vi "testpath1.vi"() -> (4 "Trajectory":T1[](array[typedef])=[{"t"=0.0, "velocity"=0.0, "acceleration"=6.476596600677185, "pose"={"Translation2d"={"x"=3.048, "y"=5.7912}, "Rotation2d"={"Theta"=0.0}}, "curvature"=0.0}, {"t"=0.17123311369028002, "velocity"=1.1090078020498375, "acceleration"=4.2961846498544, "pose"={"Translation2d"={"x"=3.1429274414869903, "y"=5.789156713424752}, "Rotation2d"={"Theta"=-0.06422251143858711}}, "curvature"=-1.352339474132374}, {"t"=0.20922733042824426, "velocity"=1.2722379727827207, "acceleration"=3.677358730976319, "pose"={"Translation2d"={"x"=3.1879379164245667, "y"=5.784637446231384}, "Rotation2d"={"Theta"=-0.14134128628704262}}, "curvature"=-2.0718634405001795}, {"t"=0.2260059617655958, "velocity"=1.3339390192249632, "acceleration"=2.69992919376837, "pose"={"Translation2d"={"x"=3.2095037093481062, "y"=5.781038434537466}, "Rotation2d"={"Theta"=-0.19076654602166596}}, "curvature"=-2.4518165820756517}, {"t"=0.2417623794212065, "velocity"=1.376480231242554, "acceleration"=1.9121141801744324, "pose"={"Translation2d"={"x"=3.2303501574005176, "y"=5.776413843665275}, "Rotation2d"={"Theta"=-0.2472086209289266}}, "curvature"=-2.8348647690280315}, {"t"=0.25676992707255936, "velocity"=1.4051763759163491, "acceleration"=1.302870542187938, "pose"={"Translation2d"={"x"=3.250421120994618, "y"=5.7706836346877255}, "Rotation2d"={"Theta"=-0.31027843147029727}}, "curvature"=-3.204804579111833}, {"t"=0.2712259317600947, "velocity"=1.4240106785814697, "acceleration"=0.8642938522151383, "pose"={"Translation2d"={"x"=3.2696708581002083, "y"=5.763782592607633}, "Rotation2d"={"Theta"=-0.3793179540434943}}, "curvature"=-3.5390528483466204}, {"t"=0.2852856144456225, "velocity"=1.436162375890667, "acceleration"=0.5888104937887121, "pose"={"Translation2d"={"x"=3.288063591012531, "y"=5.755659708693974}, "Rotation2d"={"Theta"=-0.45334831105890916}}, "curvature"=-3.8111093581327915}, {"t"=0.2990784141416015, "velocity"=1.4442837210903852, "acceleration"=0.467430338613745, "pose"={"Translation2d"={"x"=3.3055730731207307, "y"=5.746277562818135}, "Rotation2d"={"Theta"=-0.5310644010545759}}, "curvature"=-3.9951974468499536}, {"t"=0.31271519881703136, "velocity"=1.450657967968824, "acceleration"=0.47896333266736796, "pose"={"Translation2d"={"x"=3.3221821556763107, "y"=5.735611705790171}, "Rotation2d"={"Theta"=-0.6108919128048625}}, "curvature"=-4.072183097793162}, {"t"=0.3262908218291811, "velocity"=1.4571601936097591, "acceleration"=0.48871790871275284, "pose"={"Translation2d"={"x"=3.3378823545615934, "y"=5.723650041695055}, "Rotation2d"={"Theta"=-0.691106257407233}}, "curvature"=-4.034742483694034}, {"t"=0.33989122988519443, "velocity"=1.463806956592534, "acceleration"=0.6389634123631391, "pose"={"Translation2d"={"x"=3.3526734170581807, "y"=5.710392210228935}, "Rotation2d"={"Theta"=-0.7699910385979648}}, "curvature"=-3.889545372820958}, {"t"=0.3535886216760073, "velocity"=1.4725590887916666, "acceleration"=0.9100004128758293, "pose"={"Translation2d"={"x"=3.3665628886154106, "y"=5.695848969035388}, "Rotation2d"={"Theta"=-0.8459976247266188}}, "curvature"=-3.655429411840859}, {"t"=0.36742916395811687, "velocity"=1.4851539879828117, "acceleration"=1.279346026685717, "pose"={"Translation2d"={"x"=3.379565679618818, "y"=5.680041576041672}, "Rotation2d"={"Theta"=-0.9178671856268694}}, "curvature"=-3.3584701883490546}, {"t"=0.3814317421588926, "velocity"=1.5030681307673301, "acceleration"=1.7224519652606627, "pose"={"Translation2d"={"x"=3.3917036321585923, "y"=5.663001171794983}, "Rotation2d"={"Theta"=-0.9846923785837841}}, "curvature"=-3.0261374552775786}, {"t"=0.3955886938394116, "velocity"=1.5274528000115404, "acceleration"=2.2139912769151002, "pose"={"Translation2d"={"x"=3.403005086798038, "y"=5.644768161798704}, "Rotation2d"={"Theta"=-1.045917898803563}}, "curvature"=-2.682615762850822}, {"t"=0.4098690549978487, "velocity"=1.5590693950475174, "acceleration"=2.7295239699549225, "pose"={"Translation2d"={"x"=3.413504449342032, "y"=5.625391598848665}, "Rotation2d"={"Theta"=-1.1012958170019365}}, "curvature"=-2.3462802984426165}, {"t"=0.4242240484064563, "velocity"=1.5982516936448568, "acceleration"=3.2472177401001474, "pose"={"Translation2d"={"x"=3.4232417576054854, "y"=5.604928565369393}, "Rotation2d"={"Theta"=-1.1508176245777009}}, "curvature"=-2.0291930867365533}, {"t"=0.4385938505454666, "velocity"=1.6449135700723803, "acceleration"=3.749276185877941, "pose"={"Translation2d"={"x"=3.432262248181799, "y"=5.583443555750367}, "Rotation2d"={"Theta"=-1.194641984554156}}, "curvature"=-1.7378998404999786}, {"t"=0.467145646075665, "velocity"=1.7519621371178093, "acceleration"=4.698691157555746, "pose"={"Translation2d"={"x"=3.448357117149824, "y"=5.537698939493257}, "Rotation2d"={"Theta"=-1.2662953329622}}, "curvature"=-1.2393449917060648}, {"t"=0.49511151459182356, "velocity"=1.8833651162280503, "acceleration"=5.481491834882887, "pose"={"Translation2d"={"x"=3.462238461764593, "y"=5.488798473269863}, "Rotation2d"={"Theta"=-1.3187509615342337}}, "curvature"=-0.8420823071385931}, {"t"=0.5220677486425962, "velocity"=2.0311254930765528, "acceleration"=6.1297774268358065, "pose"={"Translation2d"={"x"=3.4744111411818324, "y"=5.437461941232202}, "Rotation2d"={"Theta"=-1.3543922510428046}}, "curvature"=-0.5209865526831502}, {"t"=0.5719547077588071, "velocity"=2.3369214489605827, "acceleration"=2.469114644942459, "pose"={"Translation2d"={"x"=3.4958440287769785, "y"=5.3306365296803655}, "Rotation2d"={"Theta"=-1.3817968158575638}}, "curvature"=-9.126528454248283e-16}, {"t"=0.617482683655318, "velocity"=2.4493352410012452, "acceleration"=1.7489716291390172, "pose"={"Translation2d"={"x"=3.517276916372125, "y"=5.223811118128529}, "Rotation2d"={"Theta"=-1.3543922510428048}}, "curvature"=0.5209865526831473}, {"t"=0.6388600471608528, "velocity"=2.4867236432782174, "acceleration"=-4.5602342650468595, "pose"={"Translation2d"={"x"=3.529449595789364, "y"=5.172474586090868}, "Rotation2d"={"Theta"=-1.3187509615342345}}, "curvature"=0.8420823071385926}, {"t"=0.6596998334639634, "velocity"=2.3916893357025177, "acceleration"=-10.000000000000014, "pose"={"Translation2d"={"x"=3.5433309404041333, "y"=5.123574119867473}, "Rotation2d"={"Theta"=-1.2662953329621998}}, "curvature"=1.2393449917060613}, {"t"=0.6809167339585578, "velocity"=2.1795203307565743, "acceleration"=-9.999999999999991, "pose"={"Translation2d"={"x"=3.5594258093721582, "y"=5.077829503610364}, "Rotation2d"={"Theta"=-1.1946419845541556}}, "curvature"=1.7378998404999833}, {"t"=0.6918839260254118, "velocity"=2.069848410088034, "acceleration"=-10.00000000000002, "pose"={"Translation2d"={"x"=3.568446299948472, "y"=5.056344493991338}, "Rotation2d"={"Theta"=-1.1508176245777002}}, "curvature"=2.0291930867365586}, {"t"=0.7031383604394913, "velocity"=1.9573040659472387, "acceleration"=-9.99999999999999, "pose"={"Translation2d"={"x"=3.5781836082119254, "y"=5.035881460512066}, "Rotation2d"={"Theta"=-1.1012958170019373}}, "curvature"=2.34628029844261}, {"t"=0.7147418355471609, "velocity"=1.8412693148705435, "acceleration"=-8.783912356688163, "pose"={"Translation2d"={"x"=3.5886829707559196, "y"=5.016504897562027}, "Rotation2d"={"Theta"=-1.0459178988035625}}, "curvature"=2.6826157628508227}, {"t"=0.7267353138837706, "velocity"=1.7359196523099263, "acceleration"=-7.356386910661949, "pose"={"Translation2d"={"x"=3.5999844253953652, "y"=4.998271887565748}, "Rotation2d"={"Theta"=-0.984692378583783}}, "curvature"=3.026137455277591}, {"t"=0.739111944458336, "velocity"=1.6448723691530953, "acceleration"=-5.785266152459879, "pose"={"Translation2d"={"x"=3.612122377935139, "y"=4.981231483319059}, "Rotation2d"={"Theta"=-0.9178671856268704}}, "curvature"=3.358470188349063}, {"t"=0.7518404874903905, "velocity"=1.5712343599796215, "acceleration"=-4.1137462458469605, "pose"={"Translation2d"={"x"=3.6251251689385464, "y"=4.965424090325343}, "Rotation2d"={"Theta"=-0.8459976247266192}}, "curvature"=3.6554294118408754}, {"t"=0.7648614683812988, "velocity"=1.5176693487224022, "acceleration"=-2.3761113788041133, "pose"={"Translation2d"={"x"=3.639014640495776, "y"=4.950880849131797}, "Rotation2d"={"Theta"=-0.7699910385979658}}, "curvature"=3.889545372820968}, {"t"=0.7780863251520889, "velocity"=1.4862456160662731, "acceleration"=-0.5927648597672066, "pose"={"Translation2d"={"x"=3.653805702992363, "y"=4.937623017665676}, "Rotation2d"={"Theta"=-0.6911062574072322}}, "curvature"=4.034742483694059}, {"t"=0.7914019384076868, "velocity"=1.4783525884421043, "acceleration"=0.318594910695986, "pose"={"Translation2d"={"x"=3.6695059018776464, "y"=4.92566135357056}, "Rotation2d"={"Theta"=-0.6108919128048621}}, "curvature"=4.07218309779317}, {"t"=0.8047347057336984, "velocity"=1.4826003402576653, "acceleration"=0.39202796582971616, "pose"={"Translation2d"={"x"=3.6861149844332273, "y"=4.914995496542596}, "Rotation2d"={"Theta"=-0.5310644010545743}}, "curvature"=3.995197446849954}, {"t"=0.8181096139300382, "velocity"=1.4878436783110356, "acceleration"=0.6050898214304106, "pose"={"Translation2d"={"x"=3.7036244665414264, "y"=4.905613350666757}, "Rotation2d"={"Theta"=-0.45334831105891005}}, "curvature"=3.8111093581327915}, {"t"=0.8315865754564393, "velocity"=1.4959984505544701, "acceleration"=0.9427956080909262, "pose"={"Translation2d"={"x"=3.7220171994537488, "y"=4.897490466753097}, "Rotation2d"={"Theta"=-0.3793179540434954}}, "curvature"=3.539052848346631}, {"t"=0.8451975787127834, "velocity"=1.5088308446462626, "acceleration"=1.3877862387284934, "pose"={"Translation2d"={"x"=3.74126693655934, "y"=4.890589424673006}, "Rotation2d"={"Theta"=-0.3102784314702983}}, "curvature"=3.2048045791118343}, {"t"=0.8589445083496284, "velocity"=1.527908644421045, "acceleration"=1.9216925627443424, "pose"={"Translation2d"={"x"=3.76133790015344, "y"=4.884859215695456}, "Rotation2d"={"Theta"=-0.2472086209289246}}, "curvature"=2.834864769028038}, {"t"=0.8727992700534354, "velocity"=1.554533236945846, "acceleration"=2.5272605993081534, "pose"={"Translation2d"={"x"=3.782184348205851, "y"=4.880234624823265}, "Rotation2d"={"Theta"=-0.19076654602166704}}, "curvature"=2.4518165820756592}, {"t"=0.8867067454783021, "velocity"=1.589681051622958, "acceleration"=3.1912034533747446, "pose"={"Translation2d"={"x"=3.803750141129391, "y"=4.876635613129347}, "Rotation2d"={"Theta"=-0.14134128628704148}}, "curvature"=2.0718634405001946}, {"t"=0.9143938315284367, "velocity"=1.678036176240031, "acceleration"=4.73942738227151, "pose"={"Translation2d"={"x"=3.848760616066967, "y"=4.8721163459359795}, "Rotation2d"={"Theta"=-0.06422251143858412}}, "curvature"=1.3523394741323758}, {"t"=0.96706039361214, "velocity"=1.9276455227096372, "acceleration"=3.0715111325660827, "pose"={"Translation2d"={"x"=3.9436880575539566, "y"=4.870073059360731}, "Rotation2d"={"Theta"=0.0}}, "curvature"=-5.978347474406742e-15}, {"t"=0.9914069633882024, "velocity"=2.00242628281661, "acceleration"=-9.866558396704047, "pose"={"Translation2d"={"x"=3.9915282859876635, "y"=4.870471030718632}, "Rotation2d"={"Theta"=0.02489796257300611}}, "curvature"=1.0424449028682865}, {"t"=1.0158542397991215, "velocity"=1.7612158024679117, "acceleration"=-10.0, "pose"={"Translation2d"={"x"=4.0374581515948575, "y"=4.873106215628532}, "Rotation2d"={"Theta"=0.09874992223341753}}, "curvature"=2.224603541642049}, {"t"=1.028773099528808, "velocity"=1.6320272051710467, "acceleration"=-10.00000000000001, "pose"={"Translation2d"={"x"=4.059203777534808, "y"=4.875852973414197}, "Rotation2d"={"Theta"=0.15517703568404698}}, "curvature"=2.945325833594567}, {"t"=1.0422492212162193, "velocity"=1.497265988296933, "acceleration"=-9.999999999999995, "pose"={"Translation2d"={"x"=4.079913590385775, "y"=4.879814840732562}, "Rotation2d"={"Theta"=0.22576892383844907}}, "curvature"=3.771975109233371}, {"t"=1.0564478600345162, "velocity"=1.3552796001139649, "acceleration"=-10.0, "pose"={"Translation2d"={"x"=4.099447291916161, "y"=4.8851573927805925}, "Rotation2d"={"Theta"=0.31127512742411795}}, "curvature"=4.687301631551826}, {"t"=1.0639098158850877, "velocity"=1.2806600416082508, "acceleration"=-8.960349793118844, "pose"={"Translation2d"={"x"=4.108734904396276, "y"=4.88839162423552}, "Rotation2d"={"Theta"=0.3596963482392804}}, "curvature"=5.1604774227139325}, {"t"=1.0716619724847825, "velocity"=1.2111980068239518, "acceleration"=-7.37204937958643, "pose"={"Translation2d"={"x"=4.11768515490125, "y"=4.892022365594454}, "Rotation2d"={"Theta"=0.4118045814451839}}, "curvature"=5.627208208212191}, {"t"=1.0797049284054525, "velocity"=1.1519049386189353, "acceleration"=-5.8501010886108675, "pose"={"Translation2d"={"x"=4.126286161110897, "y"=4.896063759420438}, "Rotation2d"={"Theta"=0.46741393974564627}}, "curvature"=6.070143300819135}, {"t"=1.0880171770797658, "velocity"=1.1032774436005313, "acceleration"=-4.3931111257363895, "pose"={"Translation2d"={"x"=4.134527226860072, "y"=4.900528572940315}, "Rotation2d"={"Theta"=0.5262247253095962}}, "curvature"=6.4689371688986705}, {"t"=1.0965666833417067, "velocity"=1.065718512521646, "acceleration"=-2.9947614126980446, "pose"={"Translation2d"={"x"=4.142398817255443, "y"=4.9054282266975635}, "Rotation2d"={"Theta"=0.5878142703411942}}, "curvature"=6.801867933374289}, {"t"=1.1053108923698223, "velocity"=1.0395316927396794, "acceleration"=-1.644038700543018, "pose"={"Translation2d"={"x"=4.149892533792267, "y"=4.910772823205141}, "Rotation2d"={"Theta"=0.6516384264173147}}, "curvature"=7.0482280881810375}, {"t"=1.114197959309006, "velocity"=1.024921010757345, "acceleration"=-0.3264829679038617, "pose"={"Translation2d"={"x"=4.157001089471175, "y"=4.916571175598313}, "Rotation2d"={"Theta"=0.7170462810626088}}, "curvature"=7.191153782485671}, {"t"=1.1231692479249908, "velocity"=1.021992037824076, "acceleration"=0.2202461473454793, "pose"={"Translation2d"={"x"=4.163718283914939, "y"=4.922830836287498}, "Rotation2d"={"Theta"=0.7833085290546009}}, "curvature"=7.220297530496624}, {"t"=1.1321926352252907, "velocity"=1.0239794041129733, "acceleration"=0.2613386516886456, "pose"={"Translation2d"={"x"=4.170038978485256, "y"=4.929558125611102}, "Rotation2d"={"Theta"=0.8496570437914189}}, "curvature"=7.133648349381659}, {"t"=1.1412851720405306, "velocity"=1.0263556354246974, "acceleration"=0.36975176742313487, "pose"={"Translation2d"={"x"=4.175959071399523, "y"=4.936758160488354}, "Rotation2d"={"Theta"=0.9153304525826212}}, "curvature"=6.937963941560547}, {"t"=1.1504803823584737, "velocity"=1.0297555806915843, "acceleration"=0.5404530754500246, "pose"={"Translation2d"={"x"=4.181475472847611, "y"=4.944434883072148}, "Rotation2d"={"Theta"=0.9796189350625144}}, "curvature"=6.647673983564364}, {"t"=1.1598045158588555, "velocity"=1.0347948373177722, "acceleration"=0.7676723372075956, "pose"={"Translation2d"={"x"=4.186586080108644, "y"=4.952591089401876}, "Rotation2d"={"Theta"=1.0419016817560647}}, "curvature"=6.2825755962054215}, {"t"=1.1692756134126592, "velocity"=1.0420655369128218, "acceleration"=1.0448100439943895, "pose"={"Translation2d"={"x"=4.191289752667781, "y"=4.961228458056268}, "Rotation2d"={"Theta"=1.1016723796168877}}, "curvature"=5.864961617895575}, {"t"=1.1789028252260947, "velocity"=1.0521241445111607, "acceleration"=1.3644206978494995, "pose"={"Translation2d"={"x"=4.195586287332981, "y"=4.970347578806229}, "Rotation2d"={"Theta"=1.158550959080056}}, "curvature"=5.416876643870572}, {"t"=1.1886861818206726, "velocity"=1.065472758743245, "acceleration"=1.7182932416672998, "pose"={"Translation2d"={"x"=4.199476393351792, "y"=4.979947981267677}, "Rotation2d"={"Theta"=1.2122826165113503}}, "curvature"=4.95801139300344}, {"t"=1.1986169596194587, "velocity"=1.082536747119399, "acceleration"=2.097635180915759, "pose"={"Translation2d"={"x"=4.202961667528121, "y"=4.99002816355438}, "Rotation2d"={"Theta"=1.262727036042975}}, "curvature"=4.504453400761753}, {"t"=1.2086786887623995, "velocity"=1.1036425841504771, "acceleration"=2.4933470970556573, "pose"={"Translation2d"={"x"=4.206044569339014, "y"=5.000585620930793}, "Rotation2d"={"Theta"=1.3098414998752301}}, "curvature"=4.068249389336106}, {"t"=1.2188487341307996, "velocity"=1.1290000372467017, "acceleration"=2.8963564023842063, "pose"={"Translation2d"={"x"=4.208728396051428, "y"=5.011616874464897}, "Rotation2d"={"Theta"=1.353661372079742}}, "curvature"=3.657578496396842}, {"t"=1.2394185064788306, "velocity"=1.1885774290825064, "acceleration"=3.713919348923273, "pose"={"Translation2d"={"x"=4.212916052898901, "y"=5.035082155212745}, "Rotation2d"={"Theta"=1.4318344499836884}}, "curvature"=2.929601338458617}, {"t"=1.2601460788316914, "velocity"=1.2655579611000036, "acceleration"=4.461275386160614, "pose"={"Translation2d"={"x"=4.215566826442033, "y"=5.060377779220092}, "Rotation2d"={"Theta"=1.4984049289713866}}, "curvature"=2.3317640084834035}, {"t"=1.2808006503422769, "velocity"=1.357703692591873, "acceleration"=5.095839652765746, "pose"={"Translation2d"={"x"=4.216734717164677, "y"=5.0874437665471035}, "Rotation2d"={"Theta"=1.55478349765767}}, "curvature"=1.8531035101655093}, {"t"=1.3012055233982476, "velocity"=1.4616836538201397, "acceleration"=5.595908452038135, "pose"={"Translation2d"={"x"=4.216484741399902, "y"=5.116207300782747}, "Rotation2d"={"Theta"=1.6023775716018394}}, "curvature"=1.4744007975298525}, {"t"=1.340899235076796, "velocity"=1.6838060304948936, "acceleration"=6.230746263692941, "pose"={"Translation2d"={"x"=4.212041557407635, "y"=5.178477063324598}, "Rotation2d"={"Theta"=1.6761501755710626}}, "curvature"=0.9392024761393751}, {"t"=1.378914127577943, "velocity"=1.920667179911104, "acceleration"=6.2335527791056595, "pose"={"Translation2d"={"x"=4.202947464114885, "y"=5.2463826479837765}, "Rotation2d"={"Theta"=1.7278375836964097}}, "curvature"=0.5985723564344896}, {"t"=1.4151685277805834, "velocity"=2.1466608970490815, "acceleration"=5.972100041045658, "pose"={"Translation2d"={"x"=4.190037943917913, "y"=5.318972933370419}, "Rotation2d"={"Theta"=1.762972431133745}}, "curvature"=0.37085109413942363}, {"t"=1.4497582613554434, "velocity"=2.353234246351261, "acceleration"=5.715153823531552, "pose"={"Translation2d"={"x"=4.174248291539145, "y"=5.395179436072257}, "Rotation2d"={"Theta"=1.7851143940198193}}, "curvature"=0.20712333589779897}, {"t"=1.4827014188040084, "velocity"=2.5415094586026297, "acceleration"=4.991596402415036, "pose"={"Translation2d"={"x"=4.15658813360673, "y"=5.473845651160227}, "Rotation2d"={"Theta"=1.7964066262000233}}, "curvature"=0.07732682064803718}, {"t"=1.5140101743888579, "velocity"=2.6977901303440555, "acceleration"=3.462433098634447, "pose"={"Translation2d"={"x"=4.138115948234097, "y"=5.553756392694062}, "Rotation2d"={"Theta"=1.797941459001904}}, "curvature"=-0.03890299722649509}, {"t"=1.5438194895916852, "velocity"=2.801002889949952, "acceleration"=2.28358192418938, "pose"={"Translation2d"={"x"=4.119913584599508, "y"=5.633667134227898}, "Rotation2d"={"Theta"=1.7899526357701192}}, "curvature"=-0.15806528232633305}, {"t"=1.5722131258219068, "velocity"=2.8658420844072947, "acceleration"=1.1280911880608837, "pose"={"Translation2d"={"x"=4.103060782525623, "y"=5.712333349315868}, "Rotation2d"={"Theta"=1.7718643564217582}}, "curvature"=-0.29715897337264985}, {"t"=1.5991356675412876, "velocity"=2.8962131664811297, "acceleration"=-9.20556998883836, "pose"={"Translation2d"={"x"=4.088609692059048, "y"=5.788539852017706}, "Rotation2d"={"Theta"=1.7422093760368393}}, "curvature"=-0.47809899701639796}, {"t"=1.6256014382911395, "velocity"=2.652580661534816, "acceleration"=-10.0, "pose"={"Translation2d"={"x"=4.077559393049899, "y"=5.861130137404348}, "Rotation2d"={"Theta"=1.6984091663283192}}, "curvature"=-0.7335651483582837}, {"t"=1.6527120542126659, "velocity"=2.3814745023195516, "acceleration"=-10.0, "pose"={"Translation2d"={"x"=4.070830414731352, "y"=5.929035722063526}, "Rotation2d"={"Theta"=1.6364062011238778}}, "curvature"=-1.1154107963944244}, {"t"=1.6804879513106363, "velocity"=2.1037155313398475, "acceleration"=-10.0, "pose"={"Translation2d"={"x"=4.069239255299209, "y"=5.991305484605376}, "Rotation2d"={"Theta"=1.5502007632830788}}, "curvature"=-1.704292909703093}, {"t"=1.6946526330139349, "velocity"=1.9620687143068627, "acceleration"=-10.0, "pose"={"Translation2d"={"x"=4.0705907967927235, "y"=6.02006901884102}, "Rotation2d"={"Theta"=1.4955417572753067}}, "curvature"=-2.109636818268285}, {"t"=1.7090537412581592, "velocity"=1.818057631864618, "acceleration"=-10.0, "pose"={"Translation2d"={"x"=4.073472901491444, "y"=6.047135006168031}, "Rotation2d"={"Theta"=1.4316285292429842}}, "curvature"=-2.6066526422178895}, {"t"=1.7237796290608398, "velocity"=1.670798753837812, "acceleration"=-10.000000000000009, "pose"={"Translation2d"={"x"=4.077947026190856, "y"=6.072430630175378}, "Rotation2d"={"Theta"=1.3572912194315836}}, "curvature"=-3.201603995245795}, {"t"=1.7389851361347335, "velocity"=1.5187436830988745, "acceleration"=-9.737411955646257, "pose"={"Translation2d"={"x"=4.084063348167772, "y"=6.095895910923225}, "Rotation2d"={"Theta"=1.2715767469971895}}, "curvature"=-3.8846875040570623}, {"t"=1.746841231086964, "velocity"=1.4422456501863328, "acceleration"=-8.693525280628265, "pose"={"Translation2d"={"x"=4.08774973333553, "y"=6.106927164457329}, "Rotation2d"={"Theta"=1.2242916335995968}}, "curvature"=-4.248681733504786}, {"t"=1.7548919186475858, "velocity"=1.3722567943516293, "acceleration"=-7.573674503844255, "pose"={"Translation2d"={"x"=4.091859968917197, "y"=6.117484621833742}, "Rotation2d"={"Theta"=1.1740721589970857}}, "curvature"=-4.6172536318928925}, {"t"=1.7631348285275343, "velocity"=1.3098276779563764, "acceleration"=-6.402583044036974, "pose"={"Translation2d"={"x"=4.09639680012182, "y"=6.127564804120445}, "Rotation2d"={"Theta"=1.121021538191881}}, "curvature"=-4.979251146157832}, {"t"=1.7715601144787159, "velocity"=1.2558840849841792, "acceleration"=-5.201361462476047, "pose"={"Translation2d"={"x"=4.101362117889191, "y"=6.137165206581893}, "Rotation2d"={"Theta"=1.065331019761457}}, "curvature"=-5.321029145184125}, {"t"=1.780149495611209, "velocity"=1.2112076089751114, "acceleration"=-3.9857019909796154, "pose"={"Translation2d"={"x"=4.106756934006624, "y"=6.146284327331855}, "Rotation2d"={"Theta"=1.0072891796544916}}, "curvature"=-5.627139989619832}, {"t"=1.7888758551769213, "velocity"=1.1764269402800478, "acceleration"=-2.7649783583485377, "pose"={"Translation2d"={"x"=4.1125813562257285, "y"=6.154921695986246}, "Rotation2d"={"Theta"=0.9472849671677978}}, "curvature"=-5.881543048589161}, {"t"=1.7977036043272625, "velocity"=1.1520184049264248, "acceleration"=-1.5423141829814615, "pose"={"Translation2d"={"x"=4.118834563379194, "y"=6.163077902315973}, "Rotation2d"={"Theta"=0.8858023370442392}}, "curvature"=-6.069252134391077}, {"t"=1.8065899293433723, "velocity"=1.1383128998194958, "acceleration"=-0.3155220941942261, "pose"={"Translation2d"={"x"=4.125514780497557, "y"=6.170754624899767}, "Rotation2d"={"Theta"=0.8234052766792812}}, "curvature"=-6.178180734930033}, {"t"=1.8154868927870538, "velocity"=1.135505711281776, "acceleration"=0.24470910627744785, "pose"={"Translation2d"={"x"=4.132619253925988, "y"=6.1779546597770185}, "Rotation2d"={"Theta"=0.7607136230550819}}, "curvature"=-6.200816154801577}, {"t"=1.8243675118425575, "velocity"=1.1376788796340387, "acceleration"=0.28113639026863074, "pose"={"Translation2d"={"x"=4.14014422644106, "y"=6.184681949100622}, "Rotation2d"={"Theta"=0.6983719203264055}}, "curvature"=-6.135325080865791}, {"t"=1.8332454071558555, "velocity"=1.140174779075602, "acceleration"=0.38126460611539575, "pose"={"Translation2d"={"x"=4.148084912367533, "y"=6.190941609789808}, "Rotation2d"={"Theta"=0.6370151468553518}}, "curvature"=-5.985803301665135}, {"t"=1.842148555066692, "velocity"=1.1435692342570143, "acceleration"=0.5407623442436613, "pose"={"Translation2d"={"x"=4.156435472695123, "y"=6.19673996218298}, "Rotation2d"={"Theta"=0.5772358957348409}}, "curvature"=-5.761605026760297}, {"t"=1.851098167850816, "velocity"=1.1484088478462302, "acceleration"=0.7547803531836187, "pose"={"Translation2d"={"x"=4.165188990195285, "y"=6.202084558690557}, "Rotation2d"={"Theta"=0.5195572459232708}}, "curvature"=-5.4759355108304035}, {"t"=1.8601082548048984, "velocity"=1.1552094844596477, "acceleration"=1.0179693969022292, "pose"={"Translation2d"={"x"=4.174337444537986, "y"=6.206984212447806}, "Rotation2d"={"Theta"=0.4644142421097831}}, "curvature"=-5.144063402158328}, {"t"=1.8691853505867588, "velocity"=1.1644496901783319, "acceleration"=1.3245465878706673, "pose"={"Translation2d"={"x"=4.183871687408488, "y"=6.211449025967683}, "Rotation2d"={"Theta"=0.412145081774197}}, "curvature"=-4.781547922652296}, {"t"=1.8783285252781927, "velocity"=1.176560251018176, "acceleration"=1.6684210160405477, "pose"={"Translation2d"={"x"=4.193781417624111, "y"=6.215490419793666}, "Rotation2d"={"Theta"=0.3629913658889686}}, "curvature"=-4.402790490829444}, {"t"=1.8875297493649963, "velocity"=1.1919117666578978, "acceleration"=2.0433809727929386, "pose"={"Translation2d"={"x"=4.204055156251034, "y"=6.219121161152601}, "Rotation2d"={"Theta"=0.3171055417051797}}, "curvature"=-4.020070233256811}, {"t"=1.896774632488839, "velocity"=1.2108025849288526, "acceleration"=2.4433351653567836, "pose"={"Translation2d"={"x"=4.214680221721041, "y"=6.222355392607528}, "Rotation2d"={"Theta"=0.2745631182576509}}, "curvature"=-3.6430758192368002}, {"t"=1.9153238024935424, "velocity"=1.2561244242895255, "acceleration"=3.3185049010554564, "pose"={"Translation2d"={"x"=4.236927444446259, "y"=6.227697944655556}, "Rotation2d"={"Theta"=0.19951401475255184}}, "curvature"=-2.93198664532826}, {"t"=1.933820056584235, "velocity"=1.317504334140656, "acceleration"=4.233901957263671, "pose"={"Translation2d"={"x"=4.2603966350040565, "y"=6.231659811973921}, "Rotation2d"={"Theta"=0.137466626331804}}, "curvature"=-2.298899890179479}, {"t"=1.9520324579136425, "velocity"=1.394613855775706, "acceleration"=5.173993769155555, "pose"={"Translation2d"={"x"=4.284940507922383, "y"=6.234406569759586}, "Rotation2d"={"Theta"=0.08770188039099987}}, "curvature"=-1.7466793480593512}, {"t"=1.986842242857437, "velocity"=1.574719466180544, "acceleration"=7.330345470662451, "pose"={"Translation2d"={"x"=4.336554207991923, "y"=6.237041754669483}, "Rotation2d"={"Theta"=0.022203649613225084}}, "curvature"=-0.8277745333865666}, {"t"=2.0185360873473095, "velocity"=1.807046295584759, "acceleration"=4.2458080152074125, "pose"={"Translation2d"={"x"=4.390143309352523, "y"=6.237439726027385}, "Rotation2d"={"Theta"=-2.4698950781383874e-14}}, "curvature"=-3.815788435761329e-14}, {"t"=2.0472272524369703, "velocity"=1.9288634742880806, "acceleration"=1.0486386048007321, "pose"={"Translation2d"={"x"=4.443735509762219, "y"=6.237025399682183}, "Rotation2d"={"Theta"=-0.023111687763194597}}, "curvature"=-0.8612687529609949}, {"t"=2.073842875827728, "velocity"=1.9567736444664663, "acceleration"=-9.999999999999991, "pose"={"Translation2d"={"x"=4.4953720067862015, "y"=6.234281919502013}, "Rotation2d"={"Theta"=-0.09121412756685161}}, "curvature"=-1.812232090926253}, {"t"=2.086920837778034, "velocity"=1.8259940249634075, "acceleration"=-10.0, "pose"={"Translation2d"={"x"=4.519941596714094, "y"=6.231422281259404}, "Rotation2d"={"Theta"=-0.142853118425267}}, "curvature"=-2.3779640775710726}, {"t"=2.100496514207632, "velocity"=1.6902372606674274, "acceleration"=-9.999999999999991, "pose"={"Translation2d"={"x"=4.543450100441191, "y"=6.227297597475901}, "Rotation2d"={"Theta"=-0.20706951595517584}}, "curvature"=-3.018514929278512}, {"t"=2.1146921792792663, "velocity"=1.5482806099510837, "acceleration"=-10.0, "pose"={"Translation2d"={"x"=4.565753467284166, "y"=6.22173548849439}, "Rotation2d"={"Theta"=-0.2844362355914516}}, "curvature"=-3.7245183081897935}, {"t"=2.1220895634622585, "velocity"=1.4743067681211628, "acceleration"=-9.504526862324147, "pose"={"Translation2d"={"x"=4.576413966244121, "y"=6.218368343418026}, "Rotation2d"={"Theta"=-0.3281202672351931}}, "curvature"=-4.091529876288796}, {"t"=2.129728946931762, "velocity"=1.4016980427236734, "acceleration"=-8.087405720691313, "pose"={"Translation2d"={"x"=4.5867286223244506, "y"=6.214588393510095}, "Rotation2d"={"Theta"=-0.3750828671061514}}, "curvature"=-4.457726587962087}, {"t"=2.137620002566903, "velocity"=1.3378798742377402, "acceleration"=-6.693809188303754, "pose"={"Translation2d"={"x"=4.596685195736315, "y"=6.210380915006331}, "Rotation2d"={"Theta"=-0.4251998875483632}}, "curvature"=-4.812409856452728}, {"t"=2.1457493159332444, "velocity"=1.2834638017315259, "acceleration"=-5.329606742238304, "pose"={"Translation2d"={"x"=4.606272656428732, "y"=6.205732615999336}, "Rotation2d"={"Theta"=-0.4782652371070451}}, "curvature"=-5.142699077935643}, {"t"=2.1540959506136557, "velocity"=1.2389795212638062, "acceleration"=-3.997720046989495, "pose"={"Translation2d"={"x"=4.6154811587767215, "y"=6.200631606608227}, "Rotation2d"={"Theta"=-0.5339817257639918}}, "curvature"=-5.434258292036248}, {"t"=2.1626310516406835, "velocity"=1.2048585767849769, "acceleration"=-2.697479414591349, "pose"={"Translation2d"={"x"=4.624302016269438, "y"=6.195067369148284}, "Rotation2d"={"Theta"=-0.5919579383647916}}, "curvature"=-5.672484092954958}, {"t"=2.1713181813400104, "velocity"=1.1814252232491569, "acceleration"=-1.4248404756467294, "pose"={"Translation2d"={"x"=4.6327276761983205, "y"=6.189030728300598}, "Rotation2d"={"Theta"=-0.6517131706679116}}, "curvature"=-5.844061494250866}, {"t"=2.180114497827897, "velocity"=1.168891875480618, "acceleration"=-0.17336165892091332, "pose"={"Translation2d"={"x"=4.640751694345225, "y"=6.18251382128172}, "Rotation2d"={"Theta"=-0.7126915500305057}}, "curvature"=-5.938653506639202}, {"t"=2.18897274812823, "velocity"=1.1673561945134154, "acceleration"=0.2515730993059894, "pose"={"Translation2d"={"x"=4.648368709670568, "y"=6.175510068013311}, "Rotation2d"={"Theta"=-0.7742849819238307}}, "curvature"=-5.950383323266472}, {"t"=2.1978712246817467, "velocity"=1.1695948118390853, "acceleration"=0.2953139623870331, "pose"={"Translation2d"={"x"=4.655574419001469, "y"=6.1680141412917875}, "Rotation2d"={"Theta"=-0.8358628259916795}}, "curvature"=-5.878755435370926}, {"t"=2.2068281686357123, "velocity"=1.1722399224490094, "acceleration"=0.40175171275952587, "pose"={"Translation2d"={"x"=4.662365551719884, "y"=6.160021936957975}, "Rotation2d"={"Theta"=-0.8968047161492746}}, "curvature"=-5.728773375656955}, {"t"=2.215871762692065, "velocity"=1.175873201850651, "acceleration"=0.5658375650710594, "pose"={"Translation2d"={"x"=4.668739844450756, "y"=6.151530544066752}, "Rotation2d"={"Theta"=-0.9565322033582422}}, "curvature"=-5.5102186739332355}, {"t"=2.2250243714060804, "velocity"=1.1810520916794376, "acceleration"=0.7817999513413065, "pose"={"Translation2d"={"x"=4.674696015750144, "y"=6.1425382150567}, "Rotation2d"={"Theta"=-1.014535185594998}}, "curvature"=-5.236278043907544}, {"t"=2.2343019179949044, "velocity"=1.1883052771511469, "acceleration"=1.0431227973346204, "pose"={"Translation2d"={"x"=4.680233740793372, "y"=6.133044335919754}, "Rotation2d"={"Theta"=-1.070390291884768}}, "curvature"=-4.921854667712263}, {"t"=2.243713441929392, "velocity"=1.1981226523248711, "acceleration"=1.3425872289375238, "pose"={"Translation2d"={"x"=4.685353626063164, "y"=6.123049396370849}, "Rotation2d"={"Theta"=-1.1237700816779201}}, "curvature"=-4.5819256784688}, {"t"=2.2532609597540496, "velocity"=1.2109410278243102, "acceleration"=1.6723879134618882, "pose"={"Translation2d"={"x"=4.690057184037787, "y"=6.112554960017569}, "Rotation2d"={"Theta"=-1.174443572689667}}, "curvature"=-4.2302235362806835}, {"t"=2.262939713609831, "velocity"=1.227127658790092, "acceleration"=2.0243237302703143, "pose"={"Translation2d"={"x"=4.694346807879192, "y"=6.101563634529796}, "Rotation2d"={"Theta"=-1.222269804045164}}, "curvature"=-3.878379024855448}, {"t"=2.272738836094469, "velocity"=1.2469642549715703, "acceleration"=2.3900490550749645, "pose"={"Translation2d"={"x"=4.698225746121152, "y"=6.090079041809361}, "Rotation2d"={"Theta"=-1.267186705849945}}, "curvature"=-3.5355292074324995}, {"t"=2.2926409956971012, "velocity"=1.2945313927237918, "acceleration"=3.1518207020399447, "pose"={"Translation2d"={"x"=4.704768684929782, "y"=6.065649434455436}, "Rotation2d"={"Theta"=-1.348356805225046}}, "curvature"=-2.901063627845291}, {"t"=2.3128450568015286, "velocity"=1.3582109707780066, "acceleration"=3.8735330350530868, "pose"={"Translation2d"={"x"=4.709728134319647, "y"=6.0393142642560065}, "Rotation2d"={"Theta"=-1.4185165168311715}}, "curvature"=-2.3549349277446994}, {"t"=2.333156535463395, "velocity"=1.4368881543655223, "acceleration"=4.508954594822106, "pose"={"Translation2d"={"x"=4.713158294136866, "y"=6.01113597607994}, "Rotation2d"={"Theta"=-1.4786631790472526}}, "curvature"=-1.9014375785393451}, {"t"=2.3533990911949654, "velocity"=1.5281609190423289, "acceleration"=5.0302194472129464, "pose"={"Translation2d"={"x"=4.715124620238187, "y"=5.9811903787935154}, "Rotation2d"={"Theta"=-1.529947443766078}}, "curvature"=-1.5323813127357284}, {"t"=2.39321304538764, "velocity"=1.7284338456927664, "acceleration"=5.746420515901964, "pose"={"Translation2d"={"x"=4.7149790148962545, "y"=5.91636158491433}, "Rotation2d"={"Theta"=-1.6103669248654888}}, "curvature"=-0.9953667696076589}, {"t"=2.431747494510971, "velocity"=1.9498689947040544, "acceleration"=5.92509915106607, "pose"={"Translation2d"={"x"=4.710009306139142, "y"=5.845665359789705}, "Rotation2d"={"Theta"=-1.6674653885491268}}, "curvature"=-0.6444268502130082}, {"t"=2.4687015729025767, "velocity"=2.1688255732105874, "acceleration"=5.71656233402575, "pose"={"Translation2d"={"x"=4.701061739293615, "y"=5.770091911989914}, "Rotation2d"={"Theta"=-1.7068159387324515}}, "curvature"=-0.40636135520670713}, {"t"=2.504050491035742, "velocity"=2.3708998671592014, "acceleration"=5.50122826500944, "pose"={"Translation2d"={"x"=4.689084897823565, "y"=5.690753635204437}, "Rotation2d"={"Theta"=-1.7321383059329756}}, "curvature"=-0.23415592943600302}, {"t"=2.5377742362541857, "velocity"=2.5564218875568794, "acceleration"=5.026749152333073, "pose"={"Translation2d"={"x"=4.6751037839856755, "y"=5.6088545619621675}, "Rotation2d"={"Theta"=-1.7457347670632473}}, "curvature"=-0.0977801293890419}, {"t"=2.5698261384285948, "velocity"=2.717538759642752, "acceleration"=3.4034711171348815, "pose"={"Translation2d"={"x"=4.660193899485077, "y"=5.525659817351599}, "Rotation2d"={"Theta"=-1.7488221536214548}}, "curvature"=0.02348865616992706}, {"t"=2.600334011103672, "velocity"=2.8213714231376055, "acceleration"=2.2109659300896, "pose"={"Translation2d"={"x"=4.645455326131007, "y"=5.442465072741031}, "Rotation2d"={"Theta"=-1.7417200807821853}}, "curvature"=0.14644742534608549}, {"t"=2.629420534102165, "velocity"=2.8856807345120408, "acceleration"=1.05532177828273, "pose"={"Translation2d"={"x"=4.6319868064924705, "y"=5.3605659994987604}, "Rotation2d"={"Theta"=-1.7239058478636102}}, "curvature"=0.2881434005711217}, {"t"=2.657043864118817, "velocity"=2.914832236267305, "acceleration"=-6.992140819449595, "pose"={"Translation2d"={"x"=4.620859824553896, "y"=5.281227722713285}, "Rotation2d"={"Theta"=-1.6939441226769303}}, "curvature"=0.470042292288261}, {"t"=2.6839777306885675, "velocity"=2.7265068483993438, "acceleration"=-10.000000000000007, "pose"={"Translation2d"={"x"=4.6130926863708, "y"=5.205654274913494}, "Rotation2d"={"Theta"=-1.649289411500546}}, "curvature"=0.7232762525985611}, {"t"=2.7113079148685975, "velocity"=2.4532050065990445, "acceleration"=-10.000000000000014, "pose"={"Translation2d"={"x"=4.609624600725442, "y"=5.13495804978887}, "Rotation2d"={"Theta"=-1.5859675885796558}}, "curvature"=1.0955291826446991}, {"t"=2.7252385609809466, "velocity"=2.3138985454755505, "acceleration"=-10.0, "pose"={"Translation2d"={"x"=4.609768198599568, "y"=5.101753944014012}, "Rotation2d"={"Theta"=-1.5455836843311526}}, "curvature"=1.3473789066024988}, {"t"=2.7393520691427646, "velocity"=2.172763463857369, "acceleration"=-9.999999999999986, "pose"={"Translation2d"={"x"=4.611289759782483, "y"=5.070129255909684}, "Rotation2d"={"Theta"=-1.4982245441565527}}, "curvature"=1.6570744386744032}, {"t"=2.7536746103849263, "velocity"=2.029538051435753, "acceleration"=-9.999999999999993, "pose"={"Translation2d"={"x"=4.614272897055841, "y"=5.04018365862326}, "Rotation2d"={"Theta"=-1.4428895681281102}}, "curvature"=2.0355315005356753}, {"t"=2.7682601787913192, "velocity"=1.8836823673718237, "acceleration"=-9.999999999999991, "pose"={"Translation2d"={"x"=4.618791419744651, "y"=5.012005370447193}, "Rotation2d"={"Theta"=-1.378534896890668}}, "curvature"=2.491078332554508}, {"t"=2.783205990024698, "velocity"=1.7342242550380378, "acceleration"=-10.000000000000009, "pose"={"Translation2d"={"x"=4.624908523737771, "y"=4.985670200247765}, "Rotation2d"={"Theta"=-1.3041904567429545}}, "curvature"=3.024406780560162}, {"t"=2.7986778134176538, "velocity"=1.5795060211084793, "acceleration"=-8.882568580382213, "pose"={"Translation2d"={"x"=4.632675981508393, "y"=4.961240592893841}, "Rotation2d"={"Theta"=-1.2191620970240262}}, "curvature"=3.6206919219179414}, {"t"=2.8066702480076064, "velocity"=1.5085126727390041, "acceleration"=-7.911193984009952, "pose"={"Translation2d"={"x"=4.637191449037024, "y"=4.949756000173405}, "Rotation2d"={"Theta"=-1.1725716989401087}}, "curvature"=3.9312303601515133}, {"t"=2.8148337961714707, "velocity"=1.4439292596168665, "acceleration"=-6.866866542229189, "pose"={"Translation2d"={"x"=4.642133332134536, "y"=4.938764674685631}, "Rotation2d"={"Theta"=-1.1233296337387684}}, "curvature"=4.240255681247476}, {"t"=2.8231633738637334, "velocity"=1.3867311612509696, "acceleration"=-5.769872663175095, "pose"={"Translation2d"={"x"=4.647504528830422, "y"=4.9282702383323524}, "Rotation2d"={"Theta"=-1.0715697834666007}}, "curvature"=4.537977971988079}, {"t"=2.831647225456009, "velocity"=1.3377804178702624, "acceleration"=-4.637696112704258, "pose"={"Translation2d"={"x"=4.653307071319535, "y"=4.918275298783446}, "Rotation2d"={"Theta"=-1.0175050327853297}}, "curvature"=4.812989016495026}, {"t"=2.8402663477483716, "velocity"=1.2978075479200517, "acceleration"=-3.4836594091017874, "pose"={"Translation2d"={"x"=4.659542100650238, "y"=4.908781419646502}, "Rotation2d"={"Theta"=-0.961432445963903}}, "curvature"=5.0529486299671}, {"t"=2.8489944264737344, "velocity"=1.2674018943450602, "acceleration"=-2.316287944391805, "pose"={"Translation2d"={"x"=4.666209841412529, "y"=4.89978909063645}, "Rotation2d"={"Theta"=-0.9037327110848361}}, "curvature"=5.245611332878694}, {"t"=2.8577984145005395, "velocity"=1.2470093230160013, "acceleration"=-1.1394398587684396, "pose"={"Translation2d"={"x"=4.673309576426197, "y"=4.891297697745227}, "Rotation2d"={"Theta"=-0.8448625146565251}}, "curvature"=5.380090772592848}, {"t"=2.8666397972629296, "velocity"=1.2369350990899057, "acceleration"=0.04688176129407745, "pose"={"Translation2d"={"x"=4.68083962142895, "y"=4.883305493411414}, "Rotation2d"={"Theta"=-0.7853394197847836}}, "curvature"=5.448161899394979}, {"t"=2.875476473841669, "velocity"=1.2373493780519031, "acceleration"=0.26665710039825014, "pose"={"Translation2d"={"x"=4.688797299764561, "y"=4.875809566689892}, "Rotation2d"={"Theta"=-0.725720074784665}}, "curvature"=5.445340779295286}, {"t"=2.88429554355163, "velocity"=1.2397010456089714, "acceleration"=0.3187683672546075, "pose"={"Translation2d"={"x"=4.697178917071012, "y"=4.868805813421483}, "Rotation2d"={"Theta"=-0.6665738844089412}}, "curvature"=5.371495620035246}, {"t"=2.8931191185476792, "velocity"=1.2425137222038105, "acceleration"=0.43094883309724386, "pose"={"Translation2d"={"x"=4.70597973596862, "y"=4.862288906402604}, "Rotation2d"={"Theta"=-0.6084552503474357}}, "curvature"=5.230840106245826}, {"t"=2.9019710821228784, "velocity"=1.2463284655771618, "acceleration"=0.5988377835576748, "pose"={"Translation2d"={"x"=4.715193950748202, "y"=4.85625226555492}, "Rotation2d"={"Theta"=-0.5518778106858763}}, "curvature"=5.03131266201693}, {"t"=2.9108693739877847, "velocity"=1.2516570989549916, "acceleration"=0.8175388094443056, "pose"={"Translation2d"={"x"=4.7248146620591855, "y"=4.850688028094977}, "Rotation2d"={"Theta"=-0.49729366802316216}}, "curvature"=4.7834958106091285}, {"t"=2.9198256482368925, "velocity"=1.258979200741664, "acceleration"=1.0816685830762562, "pose"={"Translation2d"={"x"=4.734833851597773, "y"=4.845587018703868}, "Rotation2d"={"Theta"=-0.44507954467127697}}, "curvature"=4.4993226623848805}, {"t"=2.928845087525624, "velocity"=1.2687352448572486, "acceleration"=1.3854520677928903, "pose"={"Translation2d"={"x"=4.7452423567950675, "y"=4.840938719696873}, "Rotation2d"={"Theta"=-0.39553048242281974}}, "curvature"=4.190826702619771}, {"t"=2.937926454595846, "velocity"=1.2813170436430736, "acceleration"=1.7228695593325305, "pose"={"Translation2d"={"x"=4.756029845505225, "y"=4.8367312411931085}, "Rotation2d"={"Theta"=-0.34886049082554704}}, "curvature"=3.8691287934167264}, {"t"=2.9562479328109226, "velocity"=1.3128825607418035, "acceleration"=2.493847148732199, "pose"={"Translation2d"={"x"=4.778694445124792, "y"=4.8295841462088145}, "Rotation2d"={"Theta"=-0.26464928277841093}}, "curvature"=3.222316485792873}, {"t"=2.9747085829510604, "velocity"=1.358920600457529, "acceleration"=3.3299467778042886, "pose"={"Translation2d"={"x"=4.802720639899954, "y"=4.824022037227305}, "Rotation2d"={"Theta"=-0.19285048592104748}}, "curvature"=2.611826396909704}, {"t"=2.9931277000968572, "velocity"=1.4202552802471746, "acceleration"=4.196602742468723, "pose"={"Translation2d"={"x"=4.8279810860838985, "y"=4.819897353443803}, "Rotation2d"={"Theta"=-0.13321073210600912}}, "curvature"=2.0619749548877087}, {"t"=3.0112991431946403, "velocity"=1.4965136081859445, "acceleration"=-9.895267674202598, "pose"={"Translation2d"={"x"=4.854327296760023, "y"=4.817037715201192}, "Rotation2d"={"Theta"=-0.08516867523010405}}, "curvature"=1.57622637937806}, {"t"=3.0544031691288542, "velocity"=1.0699877337311252, "acceleration"=-10.0, "pose"={"Translation2d"={"x"=4.909572488196385, "y"=4.814294235021023}, "Rotation2d"={"Theta"=-0.021626109447654373}}, "curvature"=0.7535046136935692}, {"t"=3.161401942501967, "velocity"=0.0, "acceleration"=-10.0, "pose"={"Translation2d"={"x"=4.966814676258997, "y"=4.813879908675812}, "Rotation2d"={"Theta"=2.3130742376130543e-14}}, "curvature"=3.346620147257001e-14}], 6 "Reverse Path?":bool)   [LabVIEW 2019]
uses:
  AutonBuilder/Typedef/Data Point.ctl
  <vilib>/Rock Robotics/WPI/ThirdParty/WPILib Extensions/Trajectory/Typedef/Trajectory State.ctl
  <vilib>/Rock Robotics/WPI/ThirdParty/WPILib Extensions/Geometry/Typedef/Pose2d.ctl
  <vilib>/Rock Robotics/WPI/ThirdParty/WPILib Extensions/Geometry/Typedef/Translation2d.ctl
  <vilib>/Rock Robotics/WPI/ThirdParty/WPILib Extensions/Geometry/Typedef/Rotation2d.ctl
panel:
  out "Total Time (s)":dbl=3.161401942501967
  out "Graph":cluster{dbl[], dbl[]}[](graph)=[{[100.5, 134.0, 134.0, 100.5, 100.5], [242.25, 242.25, 213.75, 213.75, 242.25]}, {[120.0, 155.26330935251798, 172.84028776978417, 195.5438848920863], [228.0, 191.7351598173516, 245.56849315068493, 189.52283105022832]}, {array[2202 elements], array[2202 elements]}, {array[2202 elements], array[2202 elements]}, {array[2202 elements], array[2202 elements]}]
  in  "Data Points":T5[](array[typedef])=[{"X"=120.0, "Y"=228.0, "Theta"=0.0, "Speed %"=0.0, "Disabled?"=FALSE}, {"X"=155.26330935251798, "Y"=191.7351598173516, "Theta"=0.0, "Speed %"=0.0, "Disabled?"=FALSE}, {"X"=172.84028776978417, "Y"=245.56849315068493, "Theta"=0.0, "Speed %"=0.0, "Disabled?"=FALSE}, {"X"=195.5438848920863, "Y"=189.52283105022832, "Theta"=0.0, "Speed %"=0.0, "Disabled?"=FALSE}]
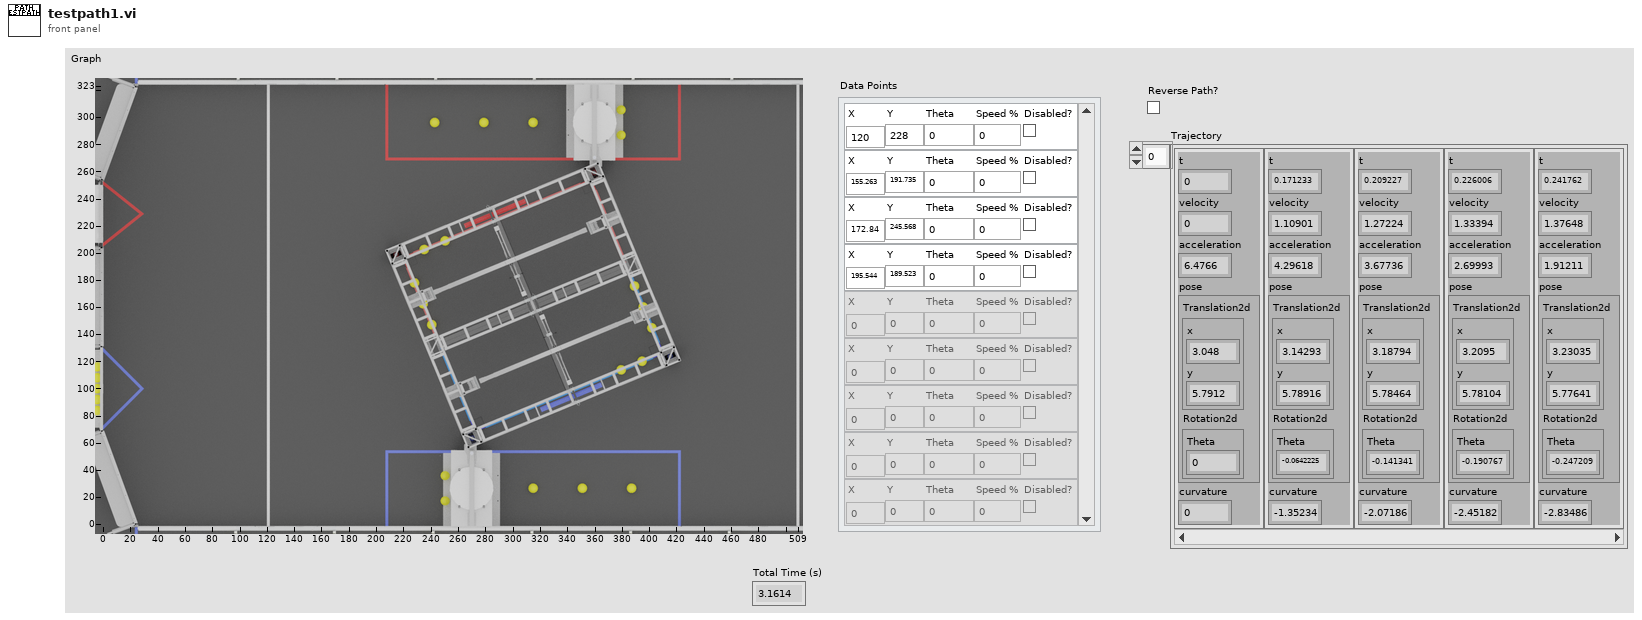
[diagram p1: front panel]
types:
  T1 = typedef "Trajectory State.ctl" = cluster{"t":dbl, "velocity":dbl, "acceleration":dbl, "pose":T2, "curvature":dbl}
  T2 = typedef "Pose2d.ctl" = cluster{"Translation2d":T3, "Rotation2d":T4}
  T3 = typedef "Translation2d.ctl" = cluster{"x":dbl, "y":dbl}
  T4 = typedef "Rotation2d.ctl" = cluster{"Theta":dbl}
  T5 = typedef "Data Point.ctl" = cluster{"X":dbl, "Y":dbl, "Theta":dbl, "Speed %":dbl, "Disabled?":bool}
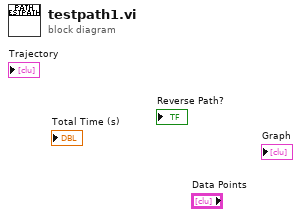
[diagram p0: block diagram]
diagram:
